vi "Command Handling Loop.vi"() -> ()   [LabVIEW 2015, in "HD44780 FPGA.lvlib"]
doc: "When using the Hitachi HD44780 VIs to control a character LCD device, you can communicate with the character LCD device either through Host VIs, or directly in LabVIEW FPGA using the FPGA VIs. No matter which VIs you use, you must first place the Command Handling Loop into the main FPGA VI."
uses:
  <vilib>/EmbeddedDisplay/Hitachi HD44780/FPGA/HD44780 FPGA.lvlib
  <vilib>/EmbeddedDisplay/Hitachi HD44780/FPGA/Internal/LCD Command.vi
  <vilib>/EmbeddedDisplay/Hitachi HD44780/FPGA/Public/Command Handler (8 Bits).vi
panel:
  in  "LCD Command":T1={"device index (-1)"=-1, "operation (0)"=0}
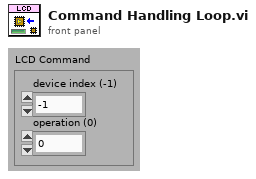
[diagram p1: front panel]
types:
  T1 = cluster{"device index (-1)":i8, "operation (0)":u32}
  T2 = cluster{"RS":refnum<k21>, "R/W":refnum<k21>, "E1":refnum<k21>, "E2":refnum<k21>, "DB0":refnum<k21>, "DB1":refnum<k21>, "DB2":refnum<k21>, "DB3":refnum<k21>, "DB4":refnum<k21>, "DB5":refnum<k21>, "DB6":refnum<k21>, "DB7":refnum<k21>}
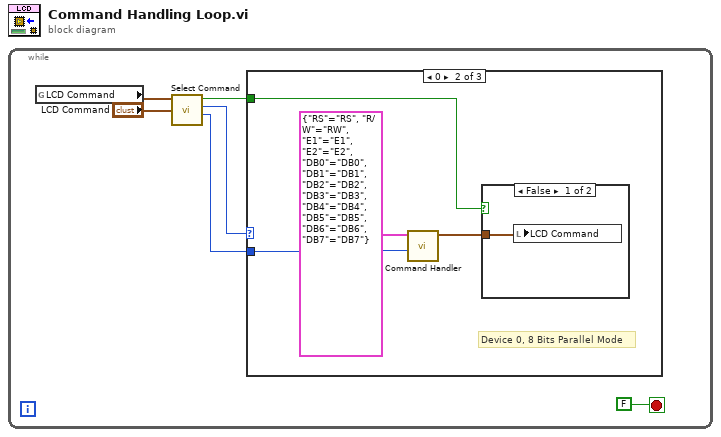
[diagram p0: block diagram]
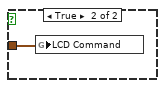
[diagram p3: hidden frame]
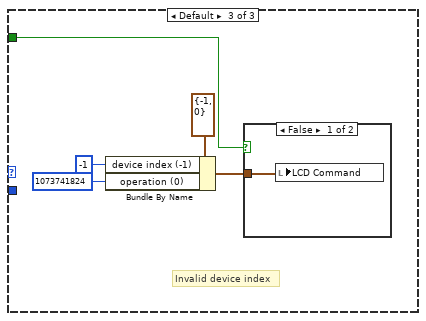
[diagram p4: hidden frame]
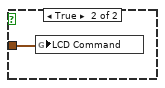
[diagram p5: hidden frame]
diagram:
  n1 = while {
    stop <- FALSE stop-if-true
    n2 = global read "LCD Command.vi" "LCD Command"() -> (w1:T1)
    n3 = call <vilib>:"Select Command.vi"("Host LCD Command"="LCD Command", "FPGA LCD Command"=w1) -> ("operation"=w3:u32, "device index"=w4:i8, "FPGA? True : False"=w2:bool)  [unwired: 7 in]
    n4 = case shown="0" w4 {
      tunnel: w3 -> [_ w10 _]
      tunnel: w2 -> [_ w9 w17]
      frame -1 {
        # "IDLE State"
      }
      frame 0 {
        # "Device 0, 8 Bits Parallel Mode"
        n5 = call-poly <vilib>:"Command Handler.vi"("operation"=w10, "device connection map in"=T2 {"RS"="RS", "R/W"="RW", "E1"="E1", "E2"="E2", "DB0"="DB0", "DB1"="DB1", "DB2"="DB2", "DB3"="DB3", "DB4"="DB4", "DB5"="DB5", "DB6"="DB6", "DB7"="DB7"}) -> ("result"=w8:T1)  [unwired: 9 in]
        n6 = case shown="False" w9 {
          tunnel: w8 -> [w11 w12]
          frame False {
            n7 = local write "LCD Command"(w11) -> ()
          }
          frame True {
            n8 = global write "LCD Command.vi" "LCD Command"(w12) -> ()
          }
        }
      }
      frame Default {
        # "Invalid device index"
        n9 = Bundle By Name(cluster=T1 {"device index (-1)"=-1, "operation (0)"=0} ("LCD Command"), "device index (-1)"=i8 -1 ("LCD_device index (-1)"), "operation (0)"=u32 1073741824 ("LCD_operation (0)")) -> (w13:T1)
        n10 = case shown="False" w17 {
          tunnel: w13 -> [w18 w19]
          frame False {
            n11 = local write "LCD Command"(w18) -> ()
          }
          frame True {
            n12 = global write "LCD Command.vi" "LCD Command"(w19) -> ()
          }
        }
      }
    }
  }
